vi "Set LakeShore 340 PID and M.vi"(4 "D":dbl, 6 "I":dbl, 7 "Manual otput":dbl, 8 "error in (no error)":errorcluster, 9 "P":dbl, 10 "Output #":i32=1, 11 "VISA Resource Name":refnum<visa-resource-name>) -> (0 "error out":errorcluster, 3 "VISA Resource Name Out":refnum<visa-resource-name>)   [LabVIEW 2024]
uses:
  Simple VISA Reader/Simple VISA Reader Driver.lvclass
  GPIB/VISA  Send Receive.vi
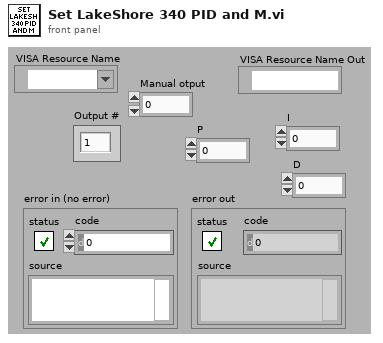
[diagram p1: front panel]
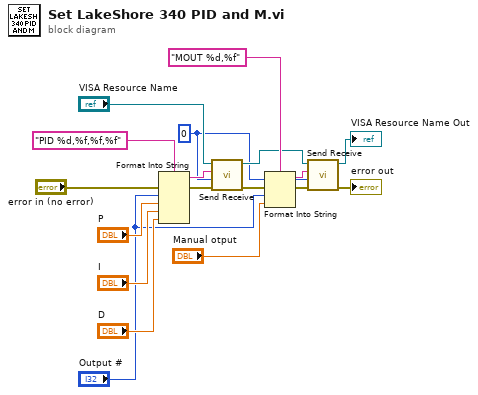
[diagram p0: block diagram]
diagram:
  w1 = 0 ("Receive count")
  n1 = Format Into String(format string="PID %d,%f,%f,%f" ("data string"), error in="error in (no error)", "Output #", "P", "I", "D") -> (resulting string=w9:string, error out=w8:errorcluster)  [unwired: 1 in]
  n2 = call-poly "Send Receive.vi"("error in (no error)"=w8, "Receive count"=w1, "data string in"=w9, "VISA Resource Name"="VISA Resource Name") -> ("error out"=w7:errorcluster, "VISA Resource Name Out"=w4:refnum<visa-resource-name>)  [unwired: 5 in, 1 out]
  n3 = Format Into String(format string="MOUT %d,%f" ("data string"), error in=w7, "Output #", "Manual otput") -> (resulting string=w2:string, error out=w6:errorcluster)  [unwired: 1 in]
  n4 = call-poly "Send Receive.vi"("error in (no error)"=w6, "Receive count"=w1, "data string in"=w2, "VISA Resource Name"=w4) -> ("error out"=→"error out":errorcluster, "VISA Resource Name Out"=→"VISA Resource Name Out":refnum<visa-resource-name>)  [unwired: 5 in, 1 out]
